vi "MotorEoTDetect.vi"(11 "output":dbl) -> (2 "result":bool)   [LabVIEW 2014]
uses:
  <vilib>/ptbypt/NI_PtbyPt.lvlib
panel:
  in  "dx/dt Tolerance":dbl=0.1 format="%#_13g"
  in  "Tolerance":dbl=0.1 format="%#_13g"
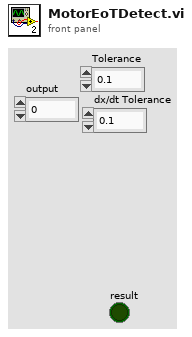
[diagram p1: front panel]
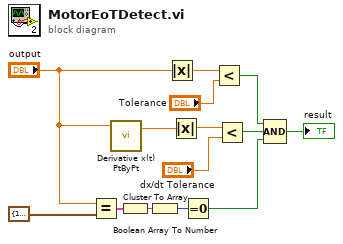
[diagram p0: block diagram]
diagram:
  n1 = Equal?(x="output", y=cluster{"output high":dbl, "output low":dbl} {"output high"=1.0, "output low"=-1.0} ("output range")) -> (x = y?=w2:cluster{"output high":bool, "output low":bool})
  n2 = call <vilib>:"Derivative x(t) PtByPt.vi"("x"="output") -> ("dx/dt"=w5:dbl)  [unwired: 3 in, 1 out]
  n3 = Cluster To Array(cluster=w2) -> (array=w3:bool[])
  n4 = Boolean Array To Number(Boolean array=w3) -> (number=w4:u32)
  n5 = Absolute Value(x="output") -> (abs(x)=w8:dbl)
  n6 = Absolute Value(x=w5) -> (abs(x)=w6:dbl)
  n7 = Equal To 0?(x=w4) -> (x = 0?=w13:bool)
  n8 = Less?(x=w8, y="Tolerance") -> (x < y?=w11:bool)
  n9 = Less?(x=w6, y="dx/dt Tolerance") -> (x < y?=w12:bool)
  n10 = Compound Arithmetic op=AND(w11, w12, w13) -> (→"result":bool)
